vi "(TestVI)Auto Tracking Set Test.vi"() -> ()   [LabVIEW 2020]
panel:
  out "출력 변수 5":dbl=131.0
  out "x-y":dbl
  out "출력 변수 4":dbl=150.0
  out "출력 변수 3":dbl=165.0
  out "출력 변수 2":dbl=134.0
  out "출력 변수":dbl=183.0
  out "결과 문자열":string="Brake Wave Set: 183Hz 0.5 Cycle\n\nTracking Range: 134Hz ~ 165Hz\nCenter Freq: 150Hz (Delta: 0)\n\nZCD_TIME Setting OK!"
  in  "ZXD":dbl=400.0
  in  "GND":dbl=100.0
  in  "Null":dbl=100.0
  in  "LRA F0":dbl=150.0
  in  "Freq.":dbl
  in  "Cycle":dbl=1.0
  in  "Scale":dbl=1.0
  in  "Voltage":dbl=1.0
  in  "PWM":dbl=48000.0
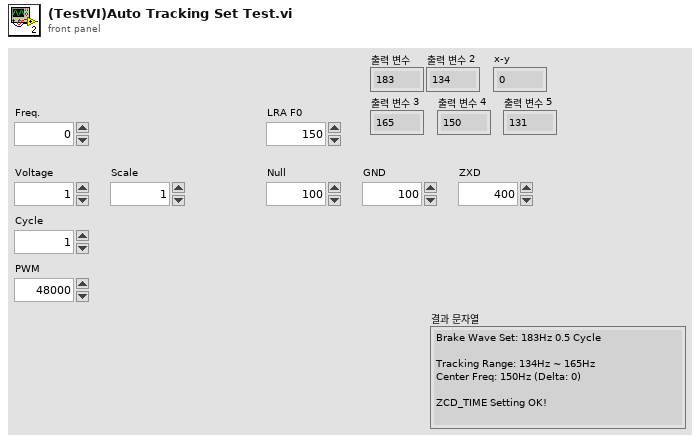
[diagram p1: front panel]
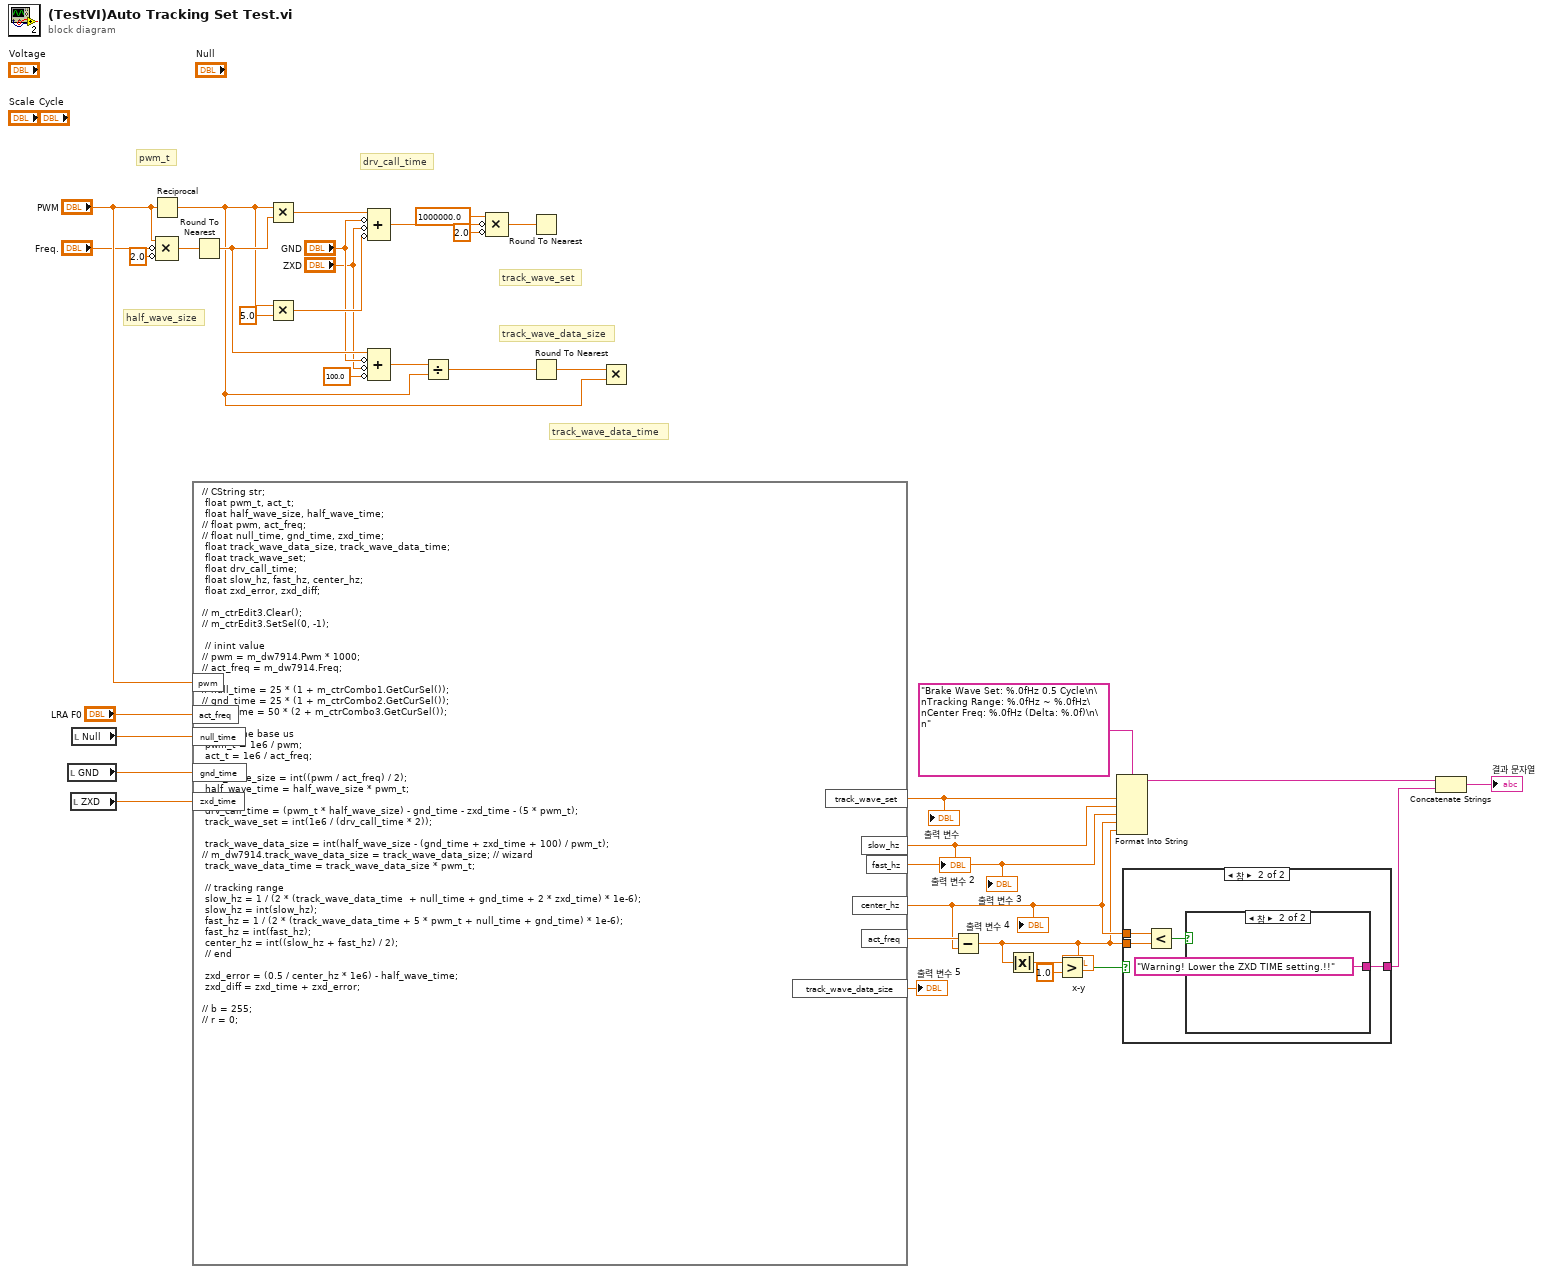
[diagram p0: block diagram]
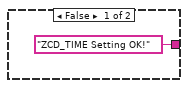
[diagram p2: hidden frame]
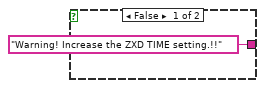
[diagram p3: hidden frame]
diagram:
  # "track_wave_data_time"
  # "track_wave_data_size"
  # "track_wave_set"
  # "drv_call_time"
  # "pwm_t"
  # "half_wave_size"
  n1 = local read "GND"() -> (w17:dbl)
  n2 = local read "ZXD"() -> (w16:dbl)
  n3 = local read "Null"() -> (w18:dbl)
  n4 = Reciprocal(x="PWM") -> (1/x=w21:dbl)
  n5 = Compound Arithmetic op=MULTIPLY("PWM", invert "Freq.", invert 2.0 ("값")) -> (w36:dbl)
  n6 = formula code="//\tCString str;\n\tfloat pwm_t, act_t;\n\tfloat half_wave_size, half_wave_time;\n//\tfloat pwm, act_freq;\n//\tfloat null_time, gnd_time, zxd_time;\n\tfloat track_wave_data_size, track_wave_data_time;\n\tfloat track_wave_set;\n\tfloat drv_call_time;\n\tfloat slow_hz, fast_hz, center_hz;\n\tfloat zxd_error, zxd_diff;\n\n//\tm_ctrEdit3.Clear();\n//\tm_ctrEdit3.SetSel(0, -1);\n\n\t// inint value\n//\tpwm = m_dw7914.Pwm * 1000;\n//\tact_freq = m_dw7914.Freq;\n\n//\tnull_time = 25 * (1 + m_ctrCombo1.GetCurSel());\n//\tgnd_time = 25 * (1 + m_ctrCombo2.GetCurSel());\n//\tzxd_time = 50 * (2 + m_ctrCombo3.GetCurSel());\n\n\t// set time base us\n\tpwm_t = 1e6 / pwm;\n\tact_t = 1e6 / act_freq;\n\n\thalf_wave_size = int((pwm / act_freq) / 2);\n\thalf_wave_time = half_wave_size * pwm_t;\n\n\tdrv_call_time = (pwm_t * half_wave_size) - gnd_time - zxd_time - (5 * pwm_t);\n\ttrack_wave_set = int(1e6 / (drv_call_time * 2));\n\n\ttrack_wave_data_size = int(half_wave_size - (gnd_time + zxd_time + 100) / pwm_t);\n//\tm_dw7914.track_wave_data_size = track_wave_data_size;\t// wizard\n\ttrack_wave_data_time = track_wave_data_size * pwm_t;\n\n\t// tracking range\n\tslow_hz = 1 / (2 * (track_wave_data_time  + null_time + gnd_time + 2 * zxd_time) * 1e-6);\n\tslow_hz = int(slow_hz);\n\tfast_hz = 1 / (2 * (track_wave_data_time + 5 * pwm_t + null_time + gnd_time) * 1e-6);\n\tfast_hz = int(fast_hz);\n\tcenter_hz = int((slow_hz + fast_hz) / 2);\n\t// end\n\n\tzxd_error = (0.5 / center_hz * 1e6) - half_wave_time;\n\tzxd_diff = zxd_time + zxd_error;\n\n//\tb = 255;\n//\tr = 0;"("pwm"="PWM", "act_freq"="LRA F0", "null_time"=w18, "gnd_time"=w17, "zxd_time"=w16) -> ("track_wave_set"=w15:dbl, "slow_hz"=w13:dbl, "fast_hz"=w12:dbl, "center_hz"=w5:dbl, "act_freq"=w11:dbl, "track_wave_data_size"=→"출력 변수 5":dbl)
  "출력 변수" <- w15
  "출력 변수 2" <- w13
  "출력 변수 3" <- w12
  "출력 변수 4" <- w5
  n7 = Round To Nearest(number=w36) -> (nearest integer value=w28:dbl)
  n8 = Multiply(x=w21, y=w28) -> (x*y=w35:dbl)
  n9 = Multiply(x=w21, y=5.0) -> (x*y=w33:dbl)
  n10 = Compound Arithmetic op=ADD(w35, invert "GND", invert "ZXD", invert w33) -> (w32:dbl)
  n11 = Compound Arithmetic op=ADD(w28, invert "GND", invert "ZXD", invert 100.0 ("값")) -> (w24:dbl)
  n12 = Divide(x=w24, y=w21) -> (x/y=w23:dbl)
  n13 = Compound Arithmetic op=MULTIPLY(1000000.0 ("x"), invert w32, invert 2.0 ("y")) -> (w29:dbl)
  n14 = Round To Nearest(number=w29) -> ()  [unwired: 1 out]
  n15 = Round To Nearest(number=w23) -> (nearest integer value=w22:dbl)
  n16 = Multiply(x=w22, y=w21) -> ()  [unwired: 1 out]
  n17 = Subtract(x=w11, y=w5) -> (x-y=w4:dbl)
  "x-y" <- w4
  n18 = Absolute Value(x=w4) -> (abs(x)=w9:dbl)
  n19 = Greater?(x=w9, y=1.0) -> (0:w6:bool)
  n20 = Format Into String(format string="Brake Wave Set: %.0fHz 0.5 Cycle\n\nTracking Range: %.0fHz ~ %.0fHz\nCenter Freq: %.0fHz (Delta: %.0f)\n\n" ("포맷 문자열"), w15, w13, w12, w5, w4) -> (resulting string=w7:string)  [unwired: 2 in, 1 out]
  n21 = case shown="참" w6 {
    tunnel: ["ZCD_TIME Setting OK!" w42] -> w3
    tunnel: w5 -> [_ w40]
    tunnel: w4 -> [_ w39]
    frame False {
    }
    frame True {
      n22 = Less?(x=w40, y=w39) -> (x < y?=w41:bool)
      n23 = case shown="참" w41 {
        tunnel: ["Warning! Increase the ZXD TIME setting.!!" "Warning! Lower the ZXD TIME setting.!!"] -> w42
        frame False {
        }
        frame True {
        }
      }
    }
  }
  n24 = Concatenate Strings(w7, w3) -> (→"결과 문자열":string)
